vi "Home Y Axis.vi"(8 "error in (no error)":errorcluster, 11 "Synchronous Home in":refnum<class "2-Axis Synchronous Home.lvclass">) -> (0 "error out":errorcluster, 3 "Synchronous Home out":refnum<class "2-Axis Synchronous Home.lvclass">)   [LabVIEW 2022 SP3, in "2-Axis Synchronous Home.lvclass"]
uses:
  2-Axis Synchronous Home.lvclass
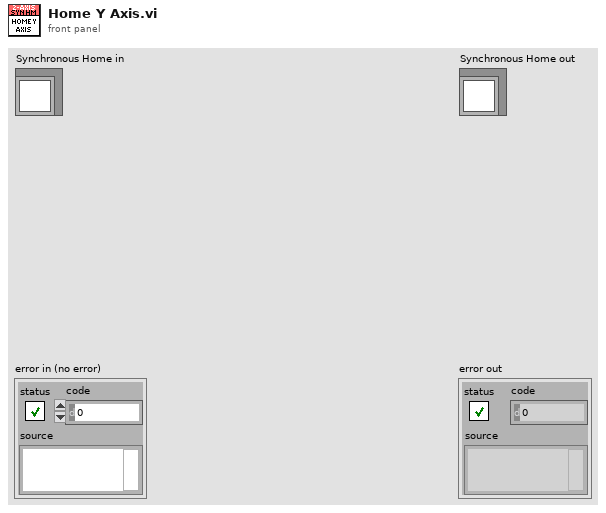
[diagram p1: front panel]
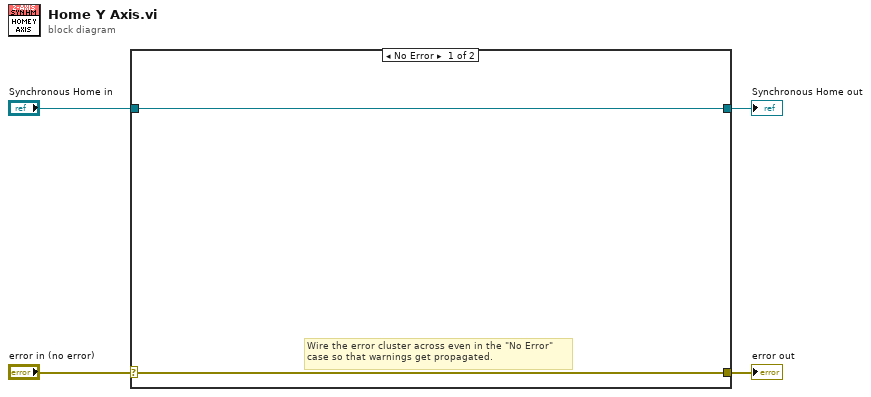
[diagram p0: block diagram]
diagram:
  n1 = case shown="No Error" "error in (no error)" {
    selector: "error in (no error)" -> [w5 w8]
    tunnel: [w5 w8] -> w3
    tunnel: [w6 w7] -> w1
    tunnel: "Synchronous Home in" -> [w6 w7]
    frame No Error {
      # "Wire the error cluster across even in the \"No Error\"\ncase so that warnings get propagated."
    }
    frame Error {
    }
  }
  "error out" <- w3
  "Synchronous Home out" <- w1
